vi "Disconnect.vi"(8 "error in (no error)":errorcluster, 11 "DPO4104 in":refnum<class "DPO4104.lvclass">) -> (0 "error out":errorcluster, 3 "DPO4104 out":refnum<class "DPO4104.lvclass">)   [LabVIEW 2018, in "DPO4104.lvlib" / "DPO4104.lvclass"]
doc: "This Override method is used finalize the communication session with the Oscope instrument."
uses:
  DPO4104.lvclass
  PPLs/Oscilloscope/Parent/Oscilloscope.lvlibp/Oscilloscope.lvclass
  <instrlib>/Tektronix DPO MSO 2000 4000 Series/Tektronix DPO MSO 2000 4000 Series.lvlib
  C:/Projects/LabVIEW/PPLs/Oscilloscope/Parent/Oscilloscope.lvlibp/Oscilloscope.lvclass
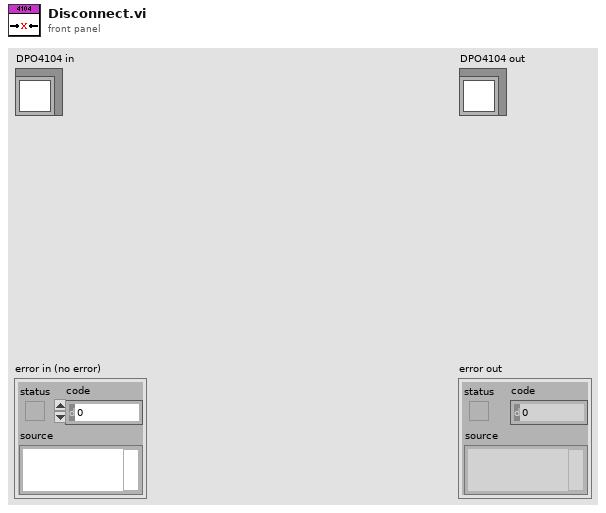
[diagram p1: front panel]
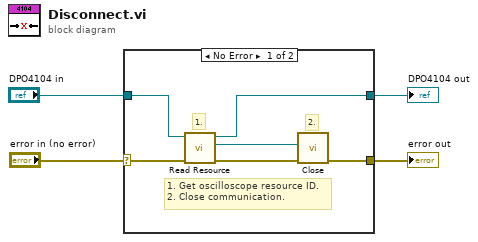
[diagram p0: block diagram]
diagram:
  n1 = case shown="No Error" "error in (no error)" {
    selector: "error in (no error)" -> [w5 w11]
    tunnel: [w10 w11] -> w4
    tunnel: [w9 w12] -> w3
    tunnel: "DPO4104 in" -> [w8 w12]
    frame No Error {
      # "2."
      # "1."
      # "1. Get oscilloscope resource ID.\n2. Close communication."
      n2 = call "Read Resource.vi"("error in (no error)"=w5, "Oscilloscope in"=w8) -> ("error out"=w7:errorcluster, "Resource"=w6:refnum<visa-resource-name>, "Oscilloscope out"=w9:refnum<class "DPO4104.lvclass">)  [unwired: 7 in]
      n3 = call <instrlib>:"Close.vi"("error in (no error)"=w7, "VISA resource name"=w6) -> ("error out"=w10:errorcluster)  [unwired: 9 in]
    }
    frame Error {
    }
  }
  "error out" <- w4
  "DPO4104 out" <- w3
